vi "ExitGlobal.vi"() -> ()   [LabVIEW 2017]
panel:
  out "StopGlobal":bool
  out "ExitGlobal":bool
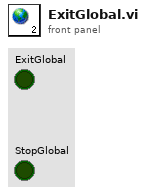
[diagram p1: front panel]
diagram:
